vi "VSS_SimulatorUDPTX.vi"(9 "Port:":u16=20011, 10 "SSL Vision Address:":string="127.0.0.1", 11 "our_robots":T1[](array[typedef])) -> ()   [LabVIEW 2018]
uses:
  Core/AI Robot.ctl
  Intel/Functions Enum.ctl
  Intel/AttackerStates.ctl
  Path Planning/RRT/PathDests.ctl
  Path Planning/RRT/PathDest.ctl
panel:
  out "error out":errorcluster
  out "Array":u8[](array[numeric]) format="%02x"
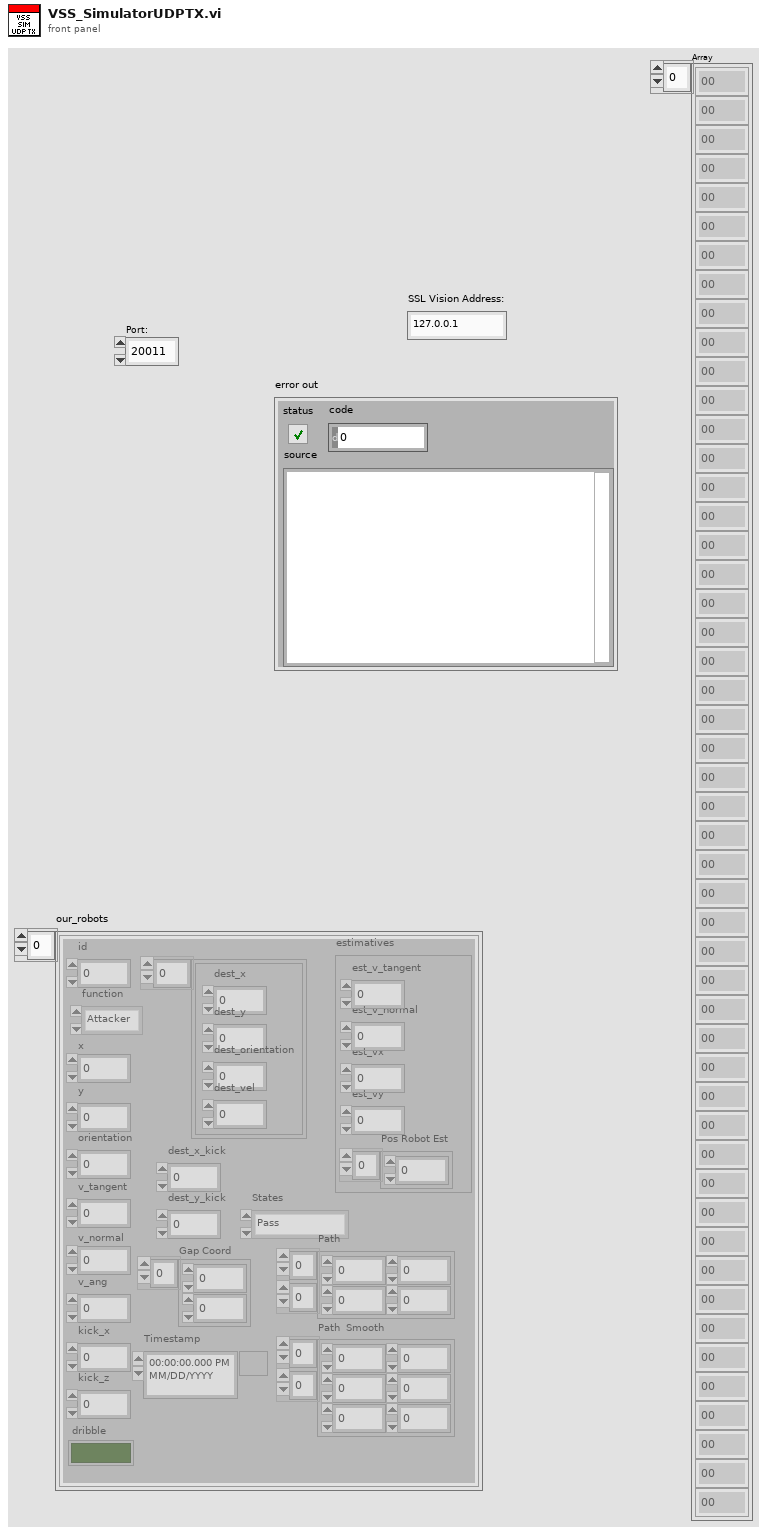
[diagram p1: front panel]
types:
  T1 = typedef "AI Robot.ctl" = cluster{"id":u32, "function":T2, "x":dbl, "y":dbl, "orientation":dbl, "v_tangent":dbl, "v_normal":dbl, "v_ang":dbl, "kick_x":dbl, "kick_z":dbl, "dribble":bool, "Timestamp":timestamp, "estimatives":cluster{"est_v_tangent":dbl, "est_v_normal":dbl, "est_vx":dbl, "est_vy":dbl, "Pos Robot Est":dbl[]}, "dest_x_kick":dbl, "dest_y_kick":dbl, "Gap Coord":dbl[], "States":T3, "Path ":dbl[][], "Path  Smooth":dbl[][], "Dest":T4}
  T2 = typedef "Functions Enum.ctl" = enum16{"Attacker", "Goalie", "Defender", "Striker", "Goto 0", "Dummy", "Kicker", "ZigZag"}
  T3 = typedef "AttackerStates.ctl" = enum16{"Pass", "GoToTangent", "BallGetting", "GoToKick", "Rotate anti-clockwise", "Rotate Clockwise", ""}
  T4 = typedef "PathDests.ctl" = T5[]
  T5 = typedef "PathDest.ctl" = cluster{"dest_x":dbl, "dest_y":dbl, "dest_orientation":dbl, "dest_vel":dbl}
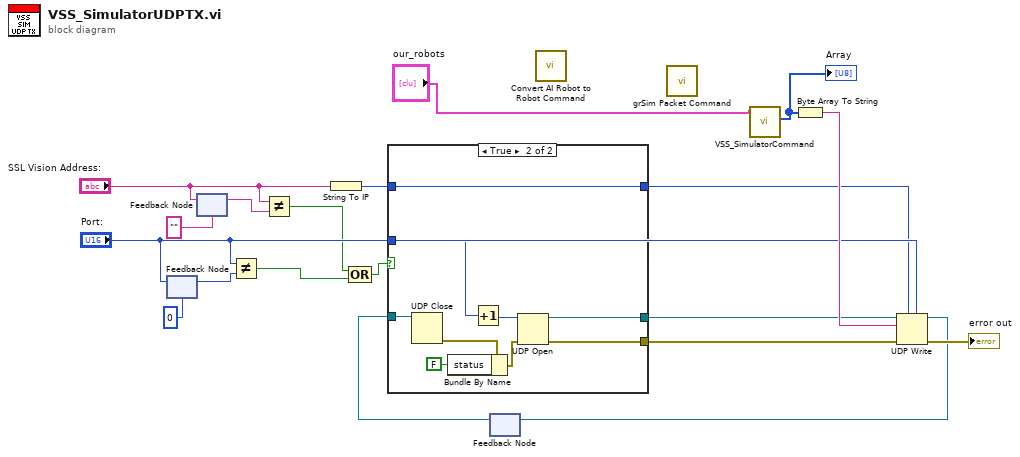
[diagram p0: block diagram]
diagram:
  n1 = feedback #1(u16 0 ("Port:")) -> (w17:u16)
  n2 = feedback-in #1("Port:") -> ()
  n3 = feedback #2("" ("SSL Vision Address:")) -> (w15:string)
  n4 = feedback-in #2("SSL Vision Address:") -> ()
  n5 = Not Equal?(x="Port:", y=w17) -> (x != y?=w13:bool)
  n6 = Not Equal?(x="SSL Vision Address:", y=w15) -> (x != y?=w14:bool)
  n7 = String To IP(1:"SSL Vision Address:") -> (0:w4:u32)
  n8 = Compound Arithmetic op=OR(w14, w13) -> (w12:bool)
  n9 = feedback #3() -> (w10:refnum<k16>)  [unwired: 1 in]
  n10 = case shown="True" w12 {
    tunnel: [_ w30] -> w18
    tunnel: [w21 w28] -> w9
    tunnel: "Port:" -> [_ w27]
    tunnel: w4 -> [w20 w25]
    tunnel: w10 -> [w21 w26]
    tunnel: [w20 w25] -> w3
    frame False {
    }
    frame True {
      n11 = UDP Close(connection ID=w26) -> (error out=w24:errorcluster)  [unwired: 1 in, 1 out]
      n12 = Bundle By Name(cluster=w24, "status"=FALSE) -> (w23:errorcluster)
      n13 = Increment(x=w27) -> (x+1=w29:u16)
      n14 = UDP Open(8:w23, 11:w29) -> (port=w28:refnum<k16>, 0:w30:errorcluster)  [unwired: 3 in, 1 out]
    }
  }
  n15 = call "Convert AI Robot to Robot Command.vi"() -> ()  [unwired: 1 in, 1 out]
  n16 = call "grSim Packet Command.vi"() -> ()  [unwired: 11 in, 1 out]
  n17 = call "VSS_SimulatorCommand.vi"("our_robots"="our_robots") -> ("Array"=w1:u8[])  [unwired: 10 in]
  "Array" <- w1
  n18 = Byte Array To String(unsigned byte array=w1) -> (string=w19:string)
  n19 = UDP Write(address=w3, port or service name="Port:", connection ID=w9, data in=w19, 8:w18) -> (error out=→"error out":errorcluster, 3:w8:refnum<k16>)  [unwired: 1 in]
  n20 = feedback-in #3(w8) -> ()
